vi "Create User Event - Stop.vi"(8 "error in (no error)":errorcluster) -> (0 "error out":errorcluster, 3 "User Event":T1)   [LabVIEW 2020, in "User Event - Stop.lvlib"]
doc: "Create a boolean user event that will be used to stop the event loop from the message handling loop."
uses:
  User Event - Stop.lvlib
  controls/Event_User.ctl
  controls/Event_Bool_Tab.ctl
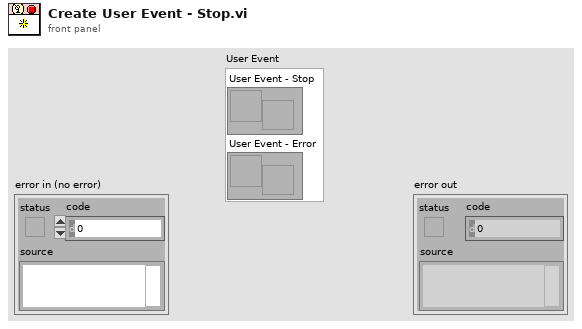
[diagram p1: front panel]
types:
  T1 = typedef "Event_User.ctl" = cluster{"User Event - Stop":refnum<user-event>, "User Event - Error":refnum<user-event>}
  T2 = typedef "Event_Bool_Tab.ctl" = cluster{"Stop Event":bool}
  T3 = cluster{"[0]":refnum<user-event>, "[1]":refnum<user-event>}
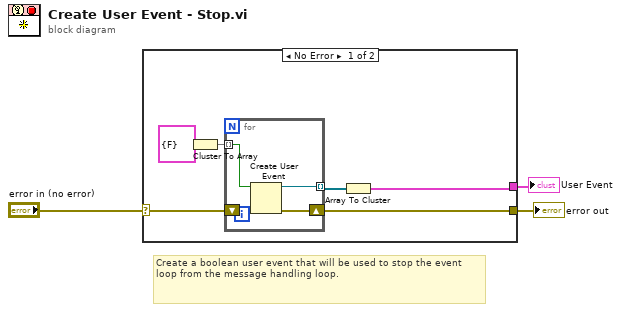
[diagram p0: block diagram]
diagram:
  # "Create a boolean user event that will be used to stop the event loop from the message handling loop."
  n1 = case shown="No Error" "error in (no error)" {
    selector: "error in (no error)" -> [w8 w14]
    tunnel: [w4 _] -> w1
    tunnel: [w9 w14] -> w3
    frame No Error {
      n2 = Cluster To Array(cluster=T2 {"Stop Event"=FALSE}) -> (array=w6:bool[])
      n3 = for {
        shift-right: [w13] -> w9
        shift-left: w8 -> [w12]
        tunnel: w6 -> [w11] mode=indexing
        tunnel: [w10] -> w5 mode=indexing
        n4 = Create User Event(user event datatype=w11, error in=w12) -> (user event=w10:refnum<user-event>, error out=w13:errorcluster)
      }
      n5 = Array To Cluster(array=w5) -> (cluster=w4:T3)
    }
    frame Error {
    }
  }
  "error out" <- w3
  "User Event" <- w1
